vi "Convert_Mala_corFiles.vi"() -> ()   [LabVIEW 2020]
panel:
  out "selected files":path[](array[path])
  in  "export":bool
  in  "Output File":path
  in  "convert":bool
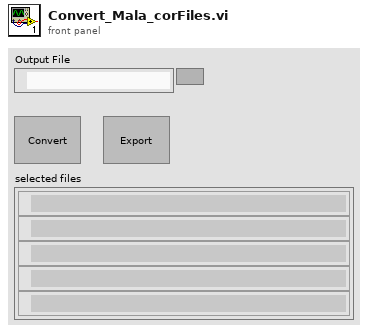
[diagram p1: front panel]
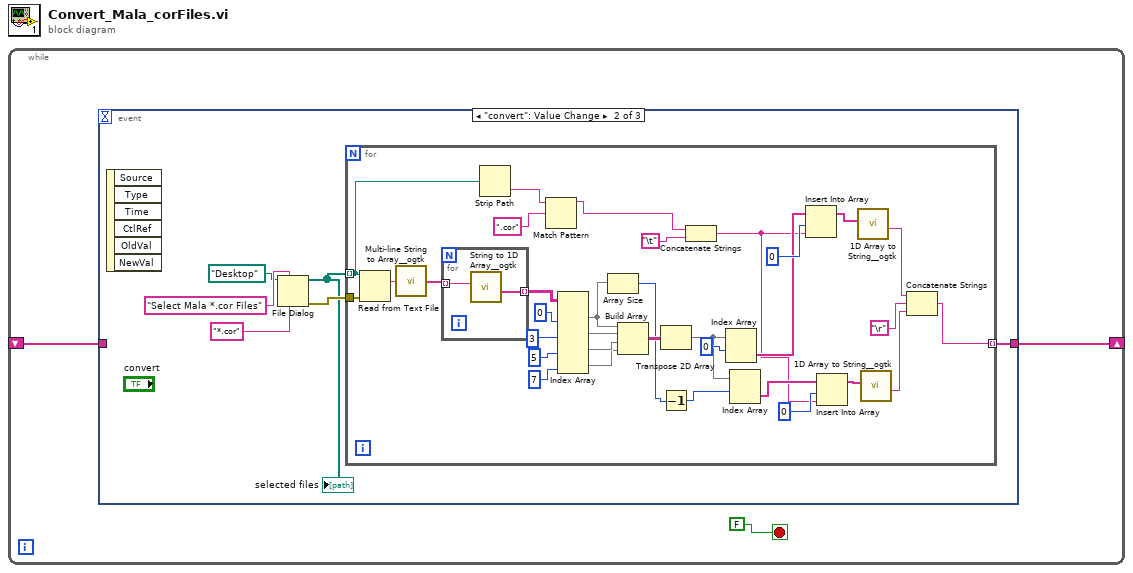
[diagram p0: block diagram]
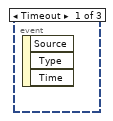
[diagram p2: hidden frame]
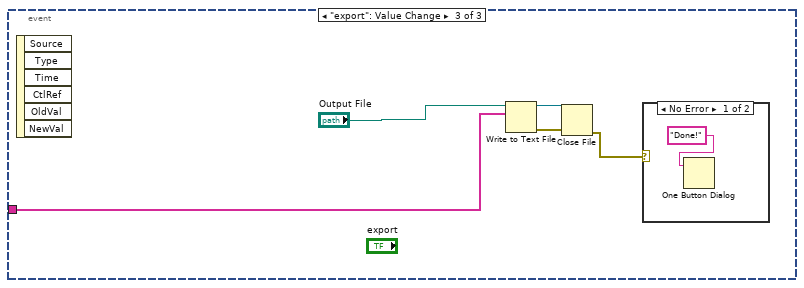
[diagram p3: hidden frame]
diagram:
  n1 = while {
    shift-right: [w2] -> _
    shift-left: _ -> [w1]
    stop <- FALSE stop-if-true
    n2 = event shown="[1] \"convert\": Value Change" {
      selector: _ -> [_ _ _]
      dyn-events: _ -> [_ _ _]
      timeout: _ -> [_ _ _]
      tunnel: [_ w4 _] -> w2
      tunnel: w1 -> [_ _ w45]
      event Timeout {
        n3 = event-data() -> ()  [unwired: 1 in, 3 out]
      }
      event "convert": Value Change {
        n4 = event-data() -> ()  [unwired: 1 in, 6 out]
        n5 = File Dialog(6:"*.cor" ("pattern (all files)"), 7:"Select Mala *.cor Files" ("button label"), 11:path "Desktop" ("start path")) -> (0:w6:errorcluster, 3:w5:path[])  [unwired: 4 in, 2 out]
        "selected files" <- w5
        n6 = for {
          tunnel: [w17] -> w4 mode=indexing
          tunnel: w6 -> [w16]
          tunnel: w5 -> [w11] mode=indexing
          n7 = Read from Text File(file (use dialog)=w11, error in=w16) -> (text=w15:string)  [unwired: 2 in, 3 out]
          n8 = call <userlib>:"Multi-line String to Array__ogtk.vi"("string"=w15) -> ("lines"=w14:string[])
          n9 = for {
            tunnel: w14 -> [w44] mode=indexing
            tunnel: [w43] -> w42 mode=indexing
            n10 = call <userlib>:"String to 1D Array__ogtk.vi"("string"=w44) -> ("Array of Strings"=w43:string[])  [unwired: 10 in]
          }
          n11 = Strip Path(path=w11) -> (name=w13:string)  [unwired: 1 out]
          n12 = Match Pattern(string=w13, regular expression=".cor") -> (before substring=w10:string)  [unwired: 1 in, 3 out]
          n13 = Index Array(array=w42, index (col) #1=0, index (col) #2=3, index (col) #3=5, index (col) #4=7) -> (element #1=w33:string[], element #2=w37:string[], element #3=w36:string[], element #4=w35:string[])  [unwired: 4 in]
          n14 = Array Size(array=w33) -> (size(s)=w30:i32)
          n15 = Build Array(w33, w37, w36, w35) -> (w34:string[][])
          n16 = Transpose 2D Array(2D array=w34) -> (transposed array=w31:string[][])
          n17 = Decrement(x=w30) -> (x-1=w29:i32)
          n18 = Concatenate Strings(w10, "\t") -> (w18:string)
          n19 = Index Array(array=w31, index (row)=0) -> (element=w27:string[])  [unwired: 1 in]
          n20 = Index Array(array=w31, index (row)=w29) -> (element=w26:string[])  [unwired: 1 in]
          n21 = Insert Into Array(array=w27, index=0, new element=w18) -> (w21:string[])
          n22 = Insert Into Array(array=w26, index=0, new element=w18) -> (w23:string[])
          n23 = call <userlib>:"1D Array to String__ogtk.vi"("Array of Strings"=w21) -> ("delimited string"=w20:string)  [unwired: 10 in]
          n24 = call <userlib>:"1D Array to String__ogtk.vi"("Array of Strings"=w23) -> ("delimited string"=w22:string)  [unwired: 10 in]
          n25 = Concatenate Strings(w20, "\r", w22) -> (w17:string)
        }
      }
      event "export": Value Change {
        n26 = event-data() -> ()  [unwired: 1 in, 6 out]
        n27 = Write to Text File(file (use dialog)="Output File", text=w45) -> (refnum out=w49:refnum<file>, error out=w48:errorcluster)  [unwired: 2 in, 1 out]
        n28 = Close File(refnum=w49, error in=w48) -> (error out=w46:errorcluster)  [unwired: 1 out]
        n29 = case shown="No Error" w46 {
          frame No Error {
            n30 = One Button Dialog(message="Done!") -> ()  [unwired: 1 in, 1 out]
          }
          frame Error {
          }
        }
      }
    }
  }
